vi "SparePinCheckMain.vi"(11 "ROI":T1={"Global Rectangle"=[536, 448, 795, 574], "Contours"=[{"Contour Type"=0, "ROI Type"=3, "Points"=[536, 448, 795, 574]}]}) -> (2 "불리언":bool=TRUE)   [LabVIEW 2014]
doc: "The Grab VI acquires images continuously and displays the images in an image control using high-level acquisition VIs. A grab is appropriate for high-speed applications in which you need to process only one image at a time."
uses:
  <vilib>/myRIO/Instrument Drivers/Onboard IO/DIO/vis/Write.vi
  <vilib>/myRIO/Instrument Drivers/Onboard IO/DIO/vis/Smart Open.vi
  <vilib>/Utility/error.llb/Error Cluster From Error Code.vi
  <vilib>/myRIO/Common/Instrument Driver Framework/myRIO v1.0/DIO/vis/myRIO v1.0 Write DIO.vi
  <vilib>/vision/driver/NI_Vision_Acquisition_Software.lvlib
  <vilib>/vision/NI_Vision_Development_Module.lvlib
panel:
  in  "BCG Values":T2={"Brightness"=180.0, "Contrast"=56.0, "Gamma"=0.89999986} {"Gamma" min=0.1 max=10 step=0.01 scale=10.0..0.1; "Contrast" min=1 max=89 step=1 scale=30.0..60.0; "Brightness" min=0 max=255 step=1 scale=0.0..255.0}
  out "최대값":u32=134
  out "불리언 2":bool=TRUE
  in  "대기시간":u32=15000
  out "웨이브폼 그래프":u32[](graph)=[39, 13, 0, 9, 0, 7, 0, 9, 0, 4, 0, 6, 0, 4, 4, 0, 4, 0, 2, 0, 4, 0, 2, 4, 0, 0, 0, 3, 8, 0, 2, 0, 2, 0, 2, 3, 0, 0, 0, 1, 3, 0, 1, 0, 3, 0, 0, 7, 0, 9, 6, 0, 23, 0, 30, 46, 0, 78, 163, 0, 404, 0, 746, 1290, 0, 1611, 2061, 0, 1985, 0, 2655, 3293, 0, 3363, 3892, 0, 4608, 3475, 0, 1735, 0, 601, 150, 0, 19, 13, 0, 1, 0, 0, 0, 0, 0, 1, 0, 1, 0, 0, 0, 0, 0, 1, 0, 0, 2, 1, 0, 1, 1, 0, 1, 2, 0, 2, 2, 0, 1, 1, 0, 0, 0, 0, 1, 0, 0, 1, 2, 0, 0, 1, 0, 0, 1, 0, 0, 1, 0, 2, 4, 0, 1, 2, 0, 2, 1, 0, 2, 1, 0, 0, 0, 0, 0, 0, 0, 1, 1, 0, 0, 0, 0, 0, 1, 0, 0, 2, 1, 0, 1, 1, 0, 0, 1, 1, 0, 1, 2, 0, 1, 2, 0, 0, 3, 0, 1, 0, 0, 0, 0, 0, 0, 1, 1, 0, 2, 1, 1, 0, 1, 1, 0, 0, 0, 0, 1, 2, 1, 0, 1, 3, 0, 1, 0, 0, 0, 0, 2, 0, 1, 0, 0, 1, 1, 1, 0, 1, 1, 0, 2, 1, 0, 0, 0, 0, 0, 1, 0, 0, 0, 1, 2, 0, 1, 1, 0, 0, 0, 0, 0, 2, 0, 1, 0, 0, 1, 134]
  in  "Camera Name":refnum<k21>="cam1" caption="IMAQdx Session"
  out "Buffer Number":u32=122
  out "Image":T3(plugin-control)
  out "Frame Rate":dbl(knob)=6.972111553784861 scale=0.0..100.0
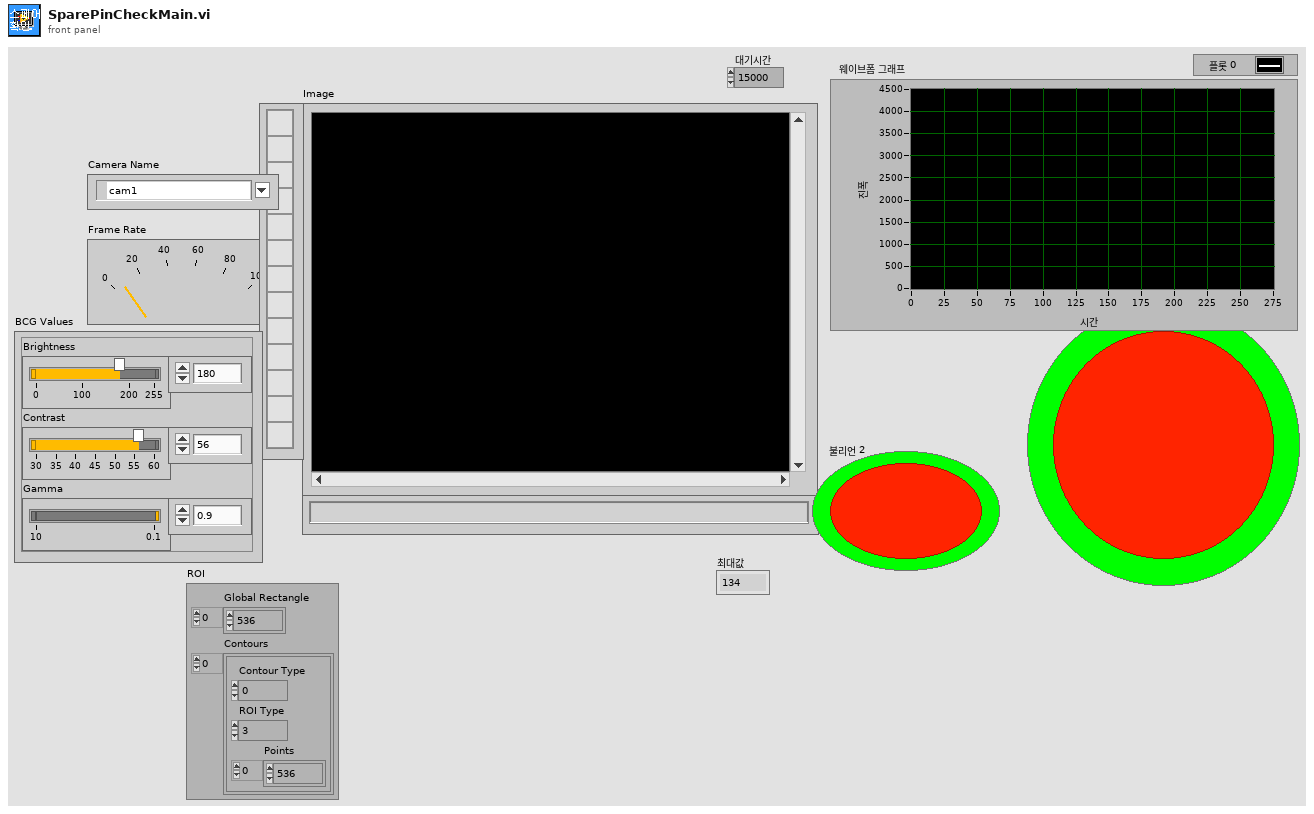
[diagram p1: front panel]
types:
  T1 = cluster{"Global Rectangle":i32[], "Contours":cluster{"Contour Type":u32, "ROI Type":u32, "Points":i32[]}[]}
  T2 = cluster{"Brightness":sgl, "Contrast":sgl, "Gamma":sgl}
  T3 = typedef "IMAQ Image.ctl" = refnum<image>
  T4 = typedef "IMAQdx.ctl" = refnum<k21>
  T5 = typedef "Image Type" = u32
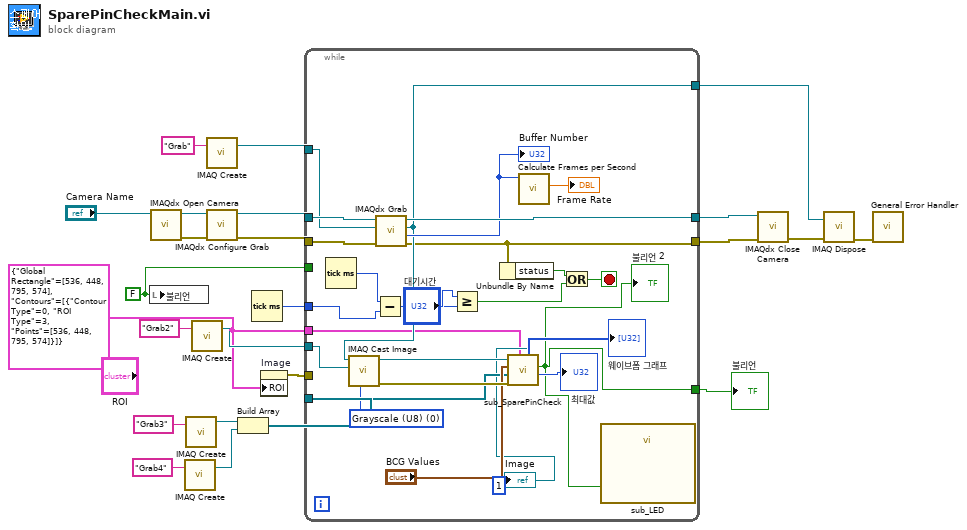
[diagram p0: block diagram]
diagram:
  w1 = T1 {"Global Rectangle"=[536, 448, 795, 574], "Contours"=[{"Contour Type"=0, "ROI Type"=3, "Points"=[536, 448, 795, 574]}]} ("ROI")
  w3 = FALSE ("불리언")
  n1 = local write "불리언"(w3) -> ()
  n2 = call <vilib>:"IMAQdx Open Camera.vi"("Session In"="Camera Name") -> ("error out"=w19:errorcluster, "Session Out"=w18:T4)  [unwired: 2 in, 7 out]
  n3 = call "IMAQ Create"("Image Name"="Grab4") -> ("New Image"=w7:T3)  [unwired: 3 in, 2 out]
  n4 = call "IMAQ Create"("Image Name"="Grab3") -> ("New Image"=w8:T3)  [unwired: 3 in, 2 out]
  n5 = call "IMAQ Create"("Image Name"="Grab2") -> ("New Image"=w11:T3)  [unwired: 3 in, 2 out]
  n6 = call "IMAQ Create"("Image Name"="Grab") -> ("New Image"=w24:T3)  [unwired: 3 in, 2 out]
  n7 = call <vilib>:"IMAQdx Configure Grab.vi"("error in"=w19, "Session In"=w18) -> ("error out"=w22:errorcluster, "Session Out"=w23:T4)  [unwired: 8 out]
  n8 = Build Array(w8, w7) -> (w6:T3[])
  n9 = Tick Count (ms)() -> (millisecond timer value=w5:u32)
  n10 = property on="Image" class="ImageControl"("ROI"=w1) -> (error out=w4:errorcluster)  [unwired: 2 in, 1 out]
  n11 = while {
    tunnel: [w47] -> w21
    tunnel: w22 -> [w49]
    tunnel: w23 -> [w50]
    tunnel: [w29] -> w20
    tunnel: w24 -> [w48]
    tunnel: [w42] -> w17
    tunnel: w11 -> [w41]
    tunnel: w6 -> [w32]
    tunnel: w5 -> [w37]
    tunnel: [w26] -> w2
    tunnel: w4 -> [_]
    tunnel: w3 -> [_]
    tunnel: w1 -> [w30]
    stop <- w25 stop-if-true
    (unwired) 1 ("인덱스")
    w39 = T5 0 items=["Grayscale (U8)", "Grayscale (I16)", "Grayscale (SGL)", "Complex (CSG)", "RGB (U32)", "HSL (U32)", "RGB (U64)", "Grayscale (U16)"] ("Image Type")
    n12 = Tick Count (ms)() -> (millisecond timer value=w38:u32)
    n13 = Subtract(x=w38, y=w37) -> (x-y=w36:u32)
    n14 = call <vilib>:"IMAQdx Grab.vi"("error in"=w49, "Image In"=w48, "Session In"=w50) -> ("error out"=w29:errorcluster, "Buffer Number Out"=w45:u32, "Image Out"=w42:T3, "Session Out"=w47:T4)  [unwired: 1 in, 4 out]
    "Buffer Number" <- w45
    n15 = call "IMAQ Cast Image"("Image Type"=w39, "Image Dst"=w41, "Image Src"=w42) -> ("error out"=w44:errorcluster, "Image Dst Out"=w43:T3)  [unwired: 7 in]
    n16 = Greater Or Equal?(x=w36, y="대기시간") -> (x >= y?=w27:bool)
    n17 = Unbundle By Name(w29) -> ("status"=w28:bool)
    n18 = call "sub_SparePinCheck.vi"("ROI"=w30, "에러 입력(에러 없음)"=w44, "추가된 배열"=w32, "BCG Values"="BCG Values", "Image Src"=w43) -> ("최대값"=→"최대값":u32, "불리언"=w26:bool, "Histogram"=→"웨이브폼 그래프":u32[], "Image Dst Out"=→"Image":T3)  [unwired: 2 in, 1 out]
    "불리언 2" <- w26
    n19 = call <vilib>:"Calculate Frames per Second.vi"("Buffer Number"=w45) -> ("Processed Frames/s"=→"Frame Rate":dbl)  [unwired: 8 in, 2 out]
    n20 = Or(x=w28, y=w27) -> (x .or. y?=w25:bool)
    n21 = call "sub_LED.vi"("LED3"=w26) -> ()  [unwired: 26 in, 1 out]
  }
  "불리언" <- w2
  n22 = call <vilib>:"IMAQdx Close Camera.vi"("error in"=w20, "Session In"=w21) -> ("error out"=w16:errorcluster)  [unwired: 9 out]
  n23 = call "IMAQ Dispose"("Image"=w17, "error in (no error)"=w16) -> ("error out"=w15:errorcluster)  [unwired: 4 in]
  n24 = call <vilib>:"General Error Handler.vi"("error in (no error)"=w15) -> ()  [unwired: 2 in, 13 out]
